vi "FGV Chiller Test.vi"(0 "Daten":T1, 7 "Chiller Konfig Daten":T2={"Bearbeiter:"="", "Gasflaschen Nr.:"="", "Accuracy"=0.0, "Sollwert"=0.0, "Messgerät:"="", "Seriennummer:"="", "Pfad:"=path "D:/IAG_Data/Log", "Textname:"="", "Einheit"="", "Expiry Date"=timestamp(0 s since 1904-01-01), "Water Concentration:"=0.0, "Componente:"=""} {"Expiry Date" format="%<%x>T"}, 11 "error in (no error)":errorcluster caption="Fehler (Eingang, kein Fehler)", 13 "Aktion":T3) -> (2 "PDF Pfad":path, 4 "Daten":T1, 8 "Chiller Konfig Daten":T2={"Bearbeiter:"="", "Gasflaschen Nr.:"="", "Accuracy"=0.0, "Sollwert"=0.0, "Messgerät:"="", "Seriennummer:"="", "Pfad:"=path "D:/IAG_Data/Log", "Textname:"="", "Einheit"="", "Expiry Date"=timestamp(0 s since 1904-01-01), "Water Concentration:"=0.0, "Componente:"=""} {"Expiry Date" format="%<%x>T"}, 15 "error out":errorcluster caption="Fehler (Ausgang)")   [LabVIEW 2020, in "EPA 1065.lvlib" / "Chiller NO2 1065-376.lvlib"]
uses:
  Chiller NO2 1065-376.lvlib
  Messdaten.ctl
  Chiller Konfig Daten.ctl
  Aktion FGV Chiller Test.ctl
  Linearisierung V2/Protokoll/Protokoll.lvlib
  Allgemein/allgemeine Sub-VIs.lvlib
panel:
  # "%"
  # "%"
  # "%"
  # "%"
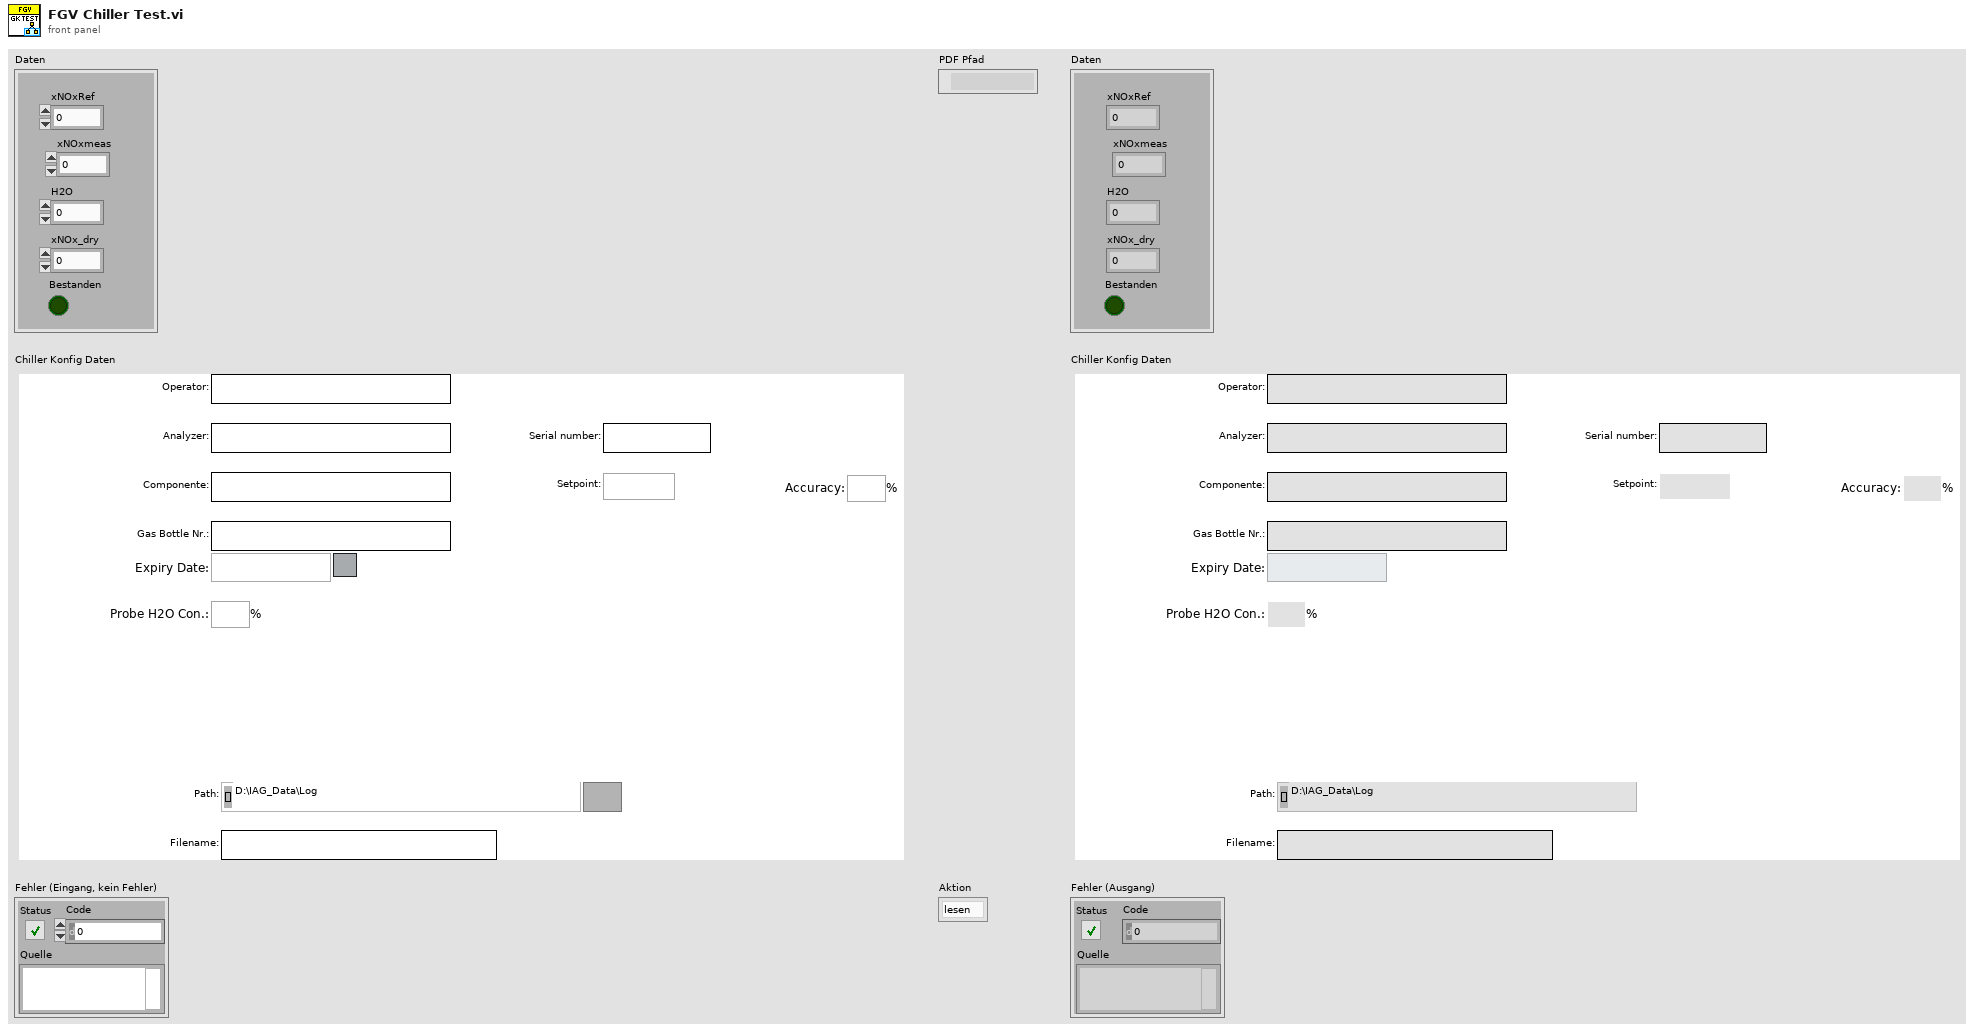
[diagram p1: front panel]
types:
  T1 = typedef "EPA 1065.lvlib/Chiller NO2 1065-376.lvlib/Messdaten.ctl" = cluster{"xNOxRef":dbl, "xNOxmeas":dbl, "H2O":dbl, "xNOx_dry":dbl, "Bestanden":bool}
  T2 = typedef "EPA 1065.lvlib/Chiller NO2 1065-376.lvlib/Chiller Konfig Daten.ctl" = cluster{"Bearbeiter:":string, "Gasflaschen Nr.:":string, "Accuracy":dbl, "Sollwert":dbl, "Messgerät:":string, "Seriennummer:":string, "Pfad:":path, "Textname:":string, "Einheit":string, "Expiry Date":timestamp, "Water Concentration:":dbl, "Componente:":string}
  T3 = typedef "EPA 1065.lvlib/Chiller NO2 1065-376.lvlib/Aktion FGV Chiller Test.ctl" = enum16{"lesen", "Konfig Daten", "Messdaten", "Resultat", "Daten löschen", "PDF einstellen", "laden", "speichern"}
  T4 = enum16{"open", "replace", "create", "open or create", "replace or create", "replace or create with confirmation"}
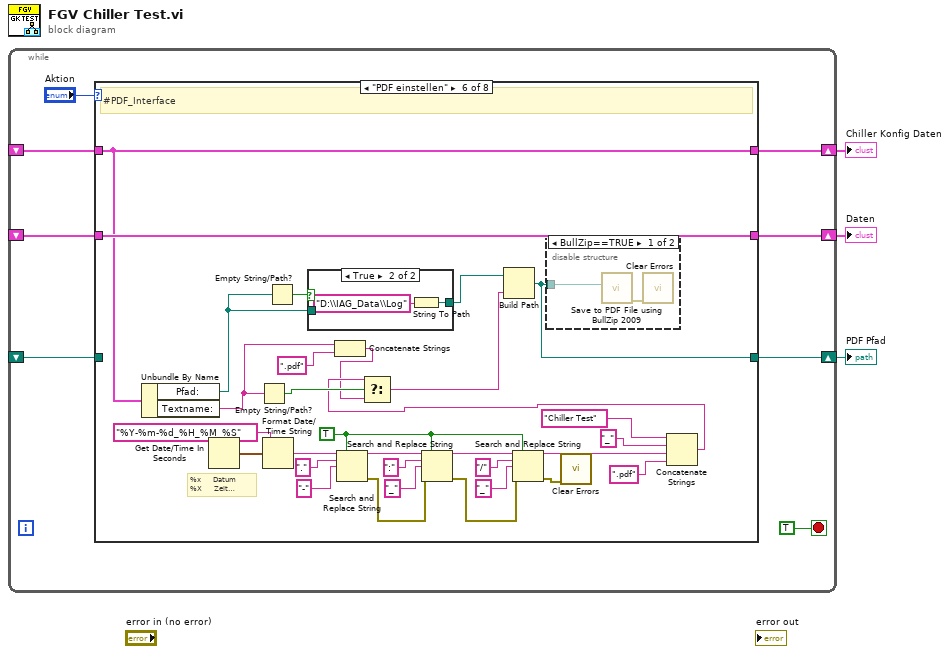
[diagram p0: block diagram]
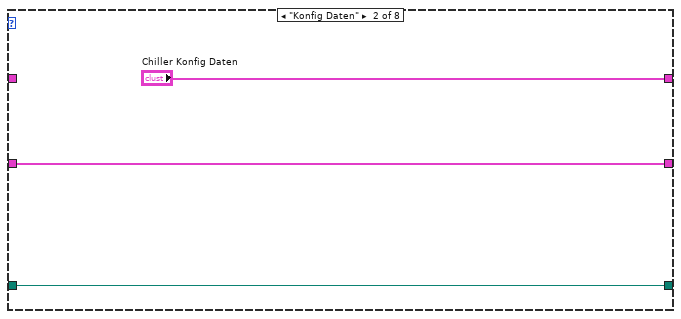
[diagram p3: hidden frame]
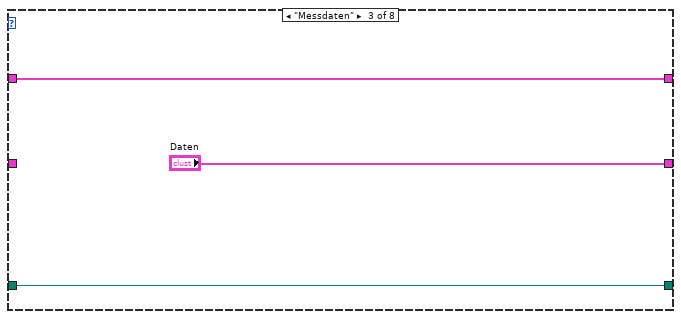
[diagram p4: hidden frame]
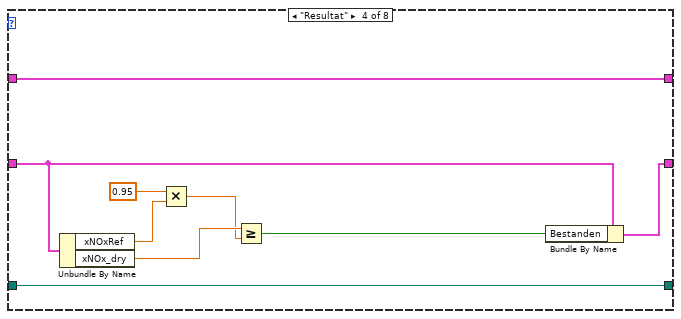
[diagram p5: hidden frame]
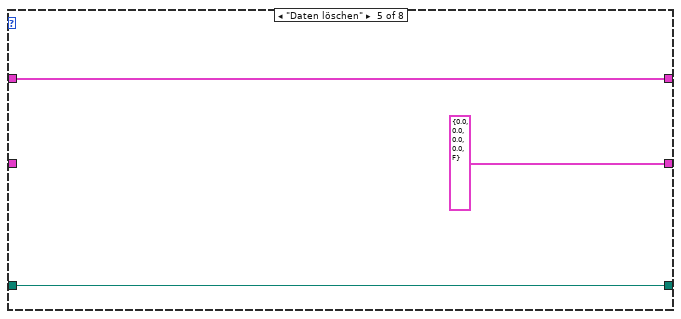
[diagram p6: hidden frame]
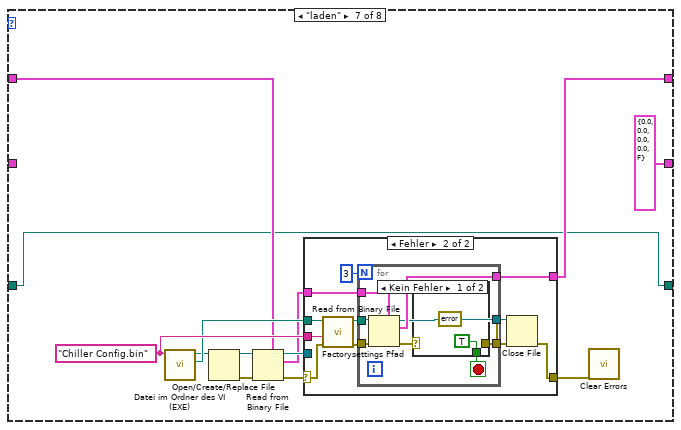
[diagram p9: hidden frame]
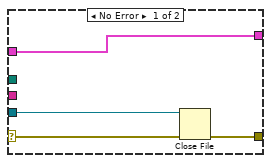
[diagram p10: hidden frame]
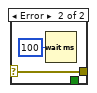
[diagram p11: hidden frame]
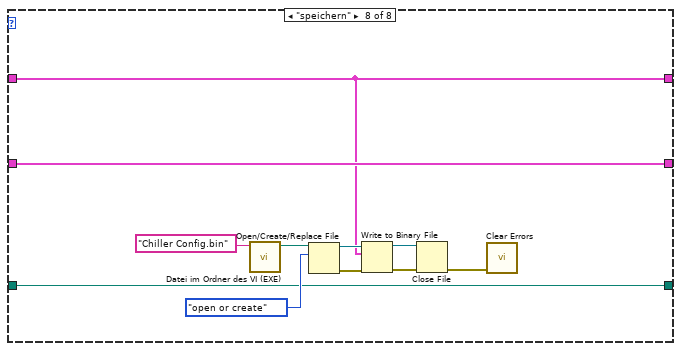
[diagram p12: hidden frame]
diagram:
  n1 = while {
    shift-right: [w9] -> w3
    shift-left: _ -> [w8]
    shift-right: [w7] -> w2
    shift-left: _ -> [w6]
    shift-right: [w5] -> w1
    shift-left: _ -> [w4]
    stop <- TRUE stop-if-true
    n2 = case shown="\"PDF einstellen\"" "Aktion" {
      tunnel: [w14 "Chiller Konfig Daten" w20 w29 w32 w62 w71 w111] -> w9
      tunnel: w8 -> [w14 _ w20 w29 w32 w62 w72 w111]
      tunnel: [w13 w16 "Daten" w24 T1 {"xNOxRef"=0.0, "xNOxmeas"=0.0, "H2O"=0.0, "xNOx_dry"=0.0, "Bestanden"=FALSE} ("Daten") w63 T1 {"xNOxRef"=0.0, "xNOxmeas"=0.0, "H2O"=0.0, "xNOx_dry"=0.0, "Bestanden"=FALSE} ("Daten") w119] -> w7
      tunnel: w6 -> [w13 w16 _ w22 _ w63 _ w119]
      tunnel: [w12 w15 w18 w21 w30 w33 w69 w109] -> w5
      tunnel: w4 -> [w12 w15 w18 w21 w30 _ w69 w109]
      frame "lesen", Default {
      }
      frame "Konfig Daten" {
      }
      frame "Messdaten" {
      }
      frame "Resultat" {
        n3 = Unbundle By Name(w22) -> ("xNOxRef"=w27:dbl, "xNOx_dry"=w26:dbl)
        n4 = Multiply(x=0.95 ("y"), y=w27) -> (x*y=w25:dbl)
        n5 = Greater Or Equal?(x=w26, y=w25) -> (x >= y?=w23:bool)
        n6 = Bundle By Name(cluster=w22, "Bestanden"=w23) -> (w24:T1)
      }
      frame "Daten löschen" {
      }
      frame "PDF einstellen" {
        w53 = TRUE ("Alle ersetzen? (F)")
        # "%x      Datum\n%X      Zeit (h:m:s)"
        # "#PDF_Interface"
        n7 = Unbundle By Name(w62) -> ("Pfad:"=w38:path, "Textname:"=w35:string)
        n8 = Get Date/Time In Seconds() -> (seconds since 1Jan1904=w61:timestamp)
        n9 = Empty String/Path?(string/path=w35) -> (empty?=w41:bool)
        n10 = Format Date/Time String(time format string (%c)="%Y-%m-%d_%H_%M_%S" ("Zeitformatierungs-String (%c)"), seconds (now)=w61) -> (date/time string=w60:string)  [unwired: 1 in]
        n11 = Empty String/Path?(string/path=w38) -> (empty?=w42:bool)
        n12 = case shown="True" w42 {
          tunnel: [w66 w67] -> w37
          tunnel: w38 -> [w66 _]
          frame False {
          }
          frame True {
            n13 = String To Path(string="D:\\IAG_Data\\Log" ("Pfad")) -> (path=w67:path)
          }
        }
        n14 = Concatenate Strings(w35, ".pdf" ("String")) -> (w34:string)
        n15 = Search and Replace String(replace all?=w53, input string=w60, search string="." ("Such-String"), replace string="-" ("String ersetzen(\"\")")) -> (result string=w59:string, error out=w56:errorcluster)  [unwired: 4 in, 2 out]
        n16 = Search and Replace String(replace all?=w53, input string=w59, search string=":" ("Such-String"), replace string="_" ("String ersetzen(\"\")"), error in=w56) -> (result string=w58:string, error out=w55:errorcluster)  [unwired: 3 in, 2 out]
        n17 = Search and Replace String(replace all?=w53, input string=w58, search string="/" ("Such-String"), replace string="_" ("String ersetzen(\"\")"), error in=w55) -> (result string=w57:string, error out=w54:errorcluster)  [unwired: 3 in, 2 out]
        n18 = call <vilib>:"Clear Errors.vi"("error in (no error)"=w54) -> ()  [unwired: 5 in, 2 out]
        n19 = Concatenate Strings("Chiller Test" ("String"), "_", w57, ".pdf" ("String")) -> (w40:string)
        n20 = Select(t=w40, s=w41, f=w34) -> (s? t:f=w39:string)
        n21 = Build Path(base path=w37, name or relative path=w39) -> (appended path=w33:path)
        n22 = disable-structure shown="BullZip==TRUE" {
          disable-tunnel: w33 -> [w65 _]
          frame condition #0 {
            n23 = call "Save to PDF File using BullZip 2009.vi"("Save PDF File Path"=w65) -> ("error out"=w64:errorcluster)  [unwired: 10 in]
            n24 = call <vilib>:"Clear Errors.vi"("error in (no error)"=w64) -> ()  [unwired: 5 in, 2 out]
          }
          frame condition #1 (active) {
          }
        }
      }
      frame "laden" {
        w79 = "Chiller Config.bin" ("Dateiname")
        n25 = call "Datei im Ordner des VI (EXE).vi"("Dateiname"=w79) -> ("Ordner des Haupt-VIs"=w78:path, "Dateipfad im Ordner des Haupt-VIs"=w75:path)  [unwired: 8 in, 1 out]
        n26 = Open/Create/Replace File(file path (use dialog)=w75) -> (refnum out=w73:refnum<file>, error out=w74:errorcluster)  [unwired: 5 in, 1 out]
        n27 = Read from Binary File(5:w72, 8:w74, 11:w73) -> (0:w81:errorcluster, 2:w76:T2, 3:w77:refnum<file>)  [unwired: 3 in, 1 out]
        n28 = case shown="Fehler" w81 {
          selector: w81 -> [w84 w88]
          tunnel: w78 -> [_ w89]
          tunnel: w76 -> [w85 w87]
          tunnel: [w85 w95] -> w71
          tunnel: [w82 w93] -> w80
          tunnel: w77 -> [w83 _]
          tunnel: w79 -> [_ w86]
          frame No Error {
            n29 = Close File(refnum=w83, error in=w84) -> (error out=w82:errorcluster)  [unwired: 1 out]
          }
          frame Error {
            n30 = call "Factorysettings Pfad.vi"("error in (no error)"=w88, "Dateiname"=w86, "Ordner des Haupt-VIs"=w89) -> ("error out"=w90:errorcluster, "Pfad Factorysettings"=w91:path)  [unwired: 7 in]
            n31 = for {
              N: 3 -> [_]
              tunnel: w90 -> [w102]
              tunnel: w91 -> [w101]
              tunnel: [w100] -> w95
              tunnel: [w99] -> w94
              tunnel: [w98] -> w92
              tunnel: w87 -> [w97]
              stop <- w103 stop-if-true
              n32 = Read from Binary File(5:w97, 8:w102, 11:w101) -> (0:w104:errorcluster, 2:w100:T2, 3:w98:refnum<file>)  [unwired: 3 in, 1 out]
              n33 = case shown="Kein Fehler" w104 {
                selector: w104 -> [_ w107]
                tunnel: [TRUE _] -> w103
                tunnel: [errorcluster {"status"=FALSE, "code"=0, "source"=""} ("error IO") w107] -> w99
                frame No Error {
                }
                frame Error {
                  n34 = Wait (ms)(milliseconds to wait=u32 100 ("Zu wartende ms")) -> ()  [unwired: 1 out]
                }
              }
            }
            n35 = Close File(refnum=w92, error in=w94) -> (error out=w93:errorcluster)  [unwired: 1 out]
          }
        }
        n36 = call <vilib>:"Clear Errors.vi"("error in (no error)"=w80) -> ()  [unwired: 5 in, 2 out]
      }
      frame "speichern" {
        n37 = call "Datei im Ordner des VI (EXE).vi"("Dateiname"="Chiller Config.bin") -> ("Dateipfad im Ordner des Haupt-VIs"=w116:path)  [unwired: 8 in, 2 out]
        n38 = Open/Create/Replace File(file path (use dialog)=w116, operation (0:open)=T4."open or create" ("Operation (0:open)")) -> (refnum out=w115:refnum<file>, error out=w117:errorcluster)  [unwired: 4 in, 1 out]
        n39 = Write to Binary File(file (use dialog)=w115, data=w111, error in=w117) -> (refnum out=w114:refnum<file>, error out=w113:errorcluster)  [unwired: 3 in, 1 out]
        n40 = Close File(refnum=w114, error in=w113) -> (error out=w112:errorcluster)  [unwired: 1 out]
        n41 = call <vilib>:"Clear Errors.vi"("error in (no error)"=w112) -> ()  [unwired: 5 in, 2 out]
      }
    }
  }
  "Chiller Konfig Daten" <- w3
  "Daten" <- w2
  "PDF Pfad" <- w1
